vi "DriveExecute.vi"(8 "error in (no error)":errorcluster) -> (0 "error out":errorcluster)   [LabVIEW 2023]
doc: "Execute for Drie\n\nClosed control loop for drive\n\ninput: \n error in (cluster)\n\noutput:\n error out (cluster)"
uses:
  <vilib>/Rock Robotics/WPI/ThirdParty/JAS_Junk/TrajLib/LinearFilter_ResetToValue.vi
  <vilib>/Rock Robotics/WPI/ThirdParty/JAS_Junk/TrajLib/LinearFilter_Calculate.vi
  DriveGlobal.vi
  <vilib>/Rock Robotics/WPI/ThirdParty/JAS_Junk/TrajLib/LinearFilter_MovingAverage.vi
  <vilib>/Rock Robotics/WPI/ThirdParty/JAS_Junk/TrajLib/LinearFilter_LowPassBW1.vi
  <vilib>/Rock Robotics/WPI/ThirdParty/JAS_Junk/TrajLib/LinearFilter_LowPassBW2.vi
  <vilib>/Rock Robotics/WPI/ThirdParty/JAS_Junk/TrajLib/LinearFilter_HighPassBW1.vi
  <vilib>/Rock Robotics/WPI/ThirdParty/JAS_Junk/TrajLib/LinearFilter_HighPassBW2.vi
  <vilib>/Rock Robotics/WPI/ThirdParty/JAS_Junk/TrajLib/Trajectory_Library.lvlib
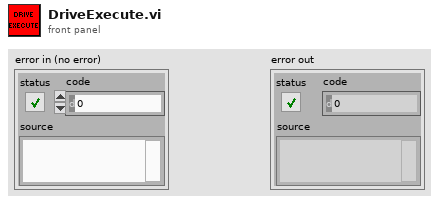
[diagram p1: front panel]
types:
  T1 = enum16{"Moving Average", "Low Pass 1st Order Butterworth", "Low Pass 2nd Order Butterworth", "High Pass 1st Order Butterworth", "High Pass 2nd Order Butterworth"}
  T2 = typedef "Trajectory_Library.lvlib/CHASSIS_SPEEDS.ctl" = cluster{"vX":dbl, "vY":dbl, "vOmega":dbl}
  T3 = typedef "ADIS16470 Device Reference.ctl" = cluster{"DevStatus":errorcluster, "Hardware Config":T4, "Calibration Complete":refnum<notifier>, "Status Reference":refnum<data-value>, "Data Reference":refnum<data-value>, "Sychronous Process VI":T8, "Cmd FIFO":refnum<k33>, "Source":T9, "Data FIFO":refnum<k33>, "Calibration Time (ms)":u32, "Data Reference":refnum<data-value>}
  T4 = typedef "ADIS16470 Hardware Configuration.ctl" = cluster{"SPI Clock Rate (Hz)":dbl, "IMU SPI Mode (3)":T5, "IMU Reset Pin":T6, "IMU SPI Bus":T7, "IMU Data Ready Pin":T6, "Stall Config":cluster{"Pow2BytesPerRead":u8, "StallTicks":u16, "CsToSclkTicks":u8}}
  T5 = typedef "WPI_SPIMode.ctl" = enum16{"Mode 0 (Clk Idle Low,Sample on Leading)", "Mode 1 (Clk Idle Low,Sample on Trailing)", "Mode 2 (Clk Idle High,Sample on Leading)", "Mode 3 (Clk Idle High,Sample on Trailing)"}
  T6 = typedef "FPGA_DIOChannel.ctl" = enum8{"DIO 0", "DIO 1", "DIO 2", "DIO 3", "DIO 4", "DIO 5", "DIO 6", "DIO 7", "DIO 8", "DIO 9", "DIO MXP 0", "DIO MXP 1", "DIO MXP 2", "DIO MXP 3", "DIO MXP 4", "DIO MXP 5", "DIO MXP 6", "DIO MXP 7", "DIO MXP 8", "DIO MXP 9", "DIO MXP 10", "DIO MXP 11", "DIO MXP 12", "DIO MXP 13", "DIO MXP 14", "DIO MXP 15", "SPI Port CS1", "SPI Port CS2", "SPI Port CS3", "SPI Port MISO", "SPI Port MOSI", "Invalid"}
  T7 = typedef "spi_bus.ctl" = enum16{"SPI On-Board, CS0", "SPI On-Board, CS1", "SPI On-Board, CS2", "SPI On-Board, CS3", "SPI MXP", "Invalid"}
  T8 = typedef "ADIS16470 Process.ctl" = refnum<vi>
  T9 = typedef "FPGA_CounterEncoderSourceConvertionLVSourceType.ctl" = cluster{"DevStatus":errorcluster, "AnalogTriggerMode?":bool, "DigitalMode":cluster{"DIO Channel":T10}, "AnalogTriggerMode":cluster{"AnalogTriggerIndex":T11, "OutputType":T12}}
  T10 = typedef "FPGA_DIODigitalSourceChannel.ctl" = enum8{"DIO 0", "DIO 1", "DIO 2", "DIO 3", "DIO 4", "DIO 5", "DIO 6", "DIO 7", "DIO 8", "DIO 9", "DIO MXP 0", "DIO MXP 1", "DIO MXP 2", "DIO MXP 3", "DIO MXP 4", "DIO MXP 5", "DIO MXP 6", "DIO MXP 7", "DIO MXP 8", "DIO MXP 9", "DIO MXP 10", "DIO MXP 11", "DIO MXP 12", "DIO MXP 13", "DIO MXP 14", "DIO MXP 15", "SPI Port CS1", "SPI Port CS2", "SPI Port CS3", "SPI Port MISO", "SPI Port MOSI", "Disabled"}
  T11 = typedef "FPGA_AnalogTriggerIndex.ctl" = enum8{"Trig 0", "Trig 1", "Trig 2", "Trig 3", "Trig 4", "Trig 5", "Trig 6", "Trig 7", "Invalid"}
  T12 = typedef "FPGA_AnalogTriggerOutType.ctl" = enum16{"InWindow", "TriggerState", "Rising", "Falling"}
  T13 = typedef "Trajectory_Library.lvlib/SWERVE_DRIVE_KINEMATICS.ctl" = cluster{"NumModules":i32, "InverseKinematics":T14, "ForwardKinematics":T14, "Modules":T15[], "PrevCoR":T15, "SavedModuleStates":T16[]}
  T14 = typedef "NI_Matrix.lvlib/RealMatrix.ctl" = dbl[][]
  T15 = typedef "Trajectory_Library.lvlib/TRANSLATION2D.ctl" = cluster{"X":dbl, "Y":dbl}
  T16 = typedef "Trajectory_Library.lvlib/SWERVE_DRIVE_MODULE_STATE.ctl" = cluster{"Speed":dbl, "Angle":T17}
  T17 = typedef "Trajectory_Library.lvlib/ROTATION2D.ctl" = cluster{"VALUE":dbl, "COS":dbl, "SIN":dbl}
  T18 = typedef "Trajectory_Library.lvlib/SWERVE_DRIVE_MODULE_POSITION.ctl" = cluster{"Distance":dbl, "Angle":T17, "P":bool}
  T19 = typedef "ADIS16470 Data.ctl" = cluster{"XAngle":dbl, "YAngle":dbl, "ZAngle":dbl}
  T20 = typedef "ADIS16470 Status.ctl" = cluster{"Calibrated?":bool, "IMU Detected?":bool}
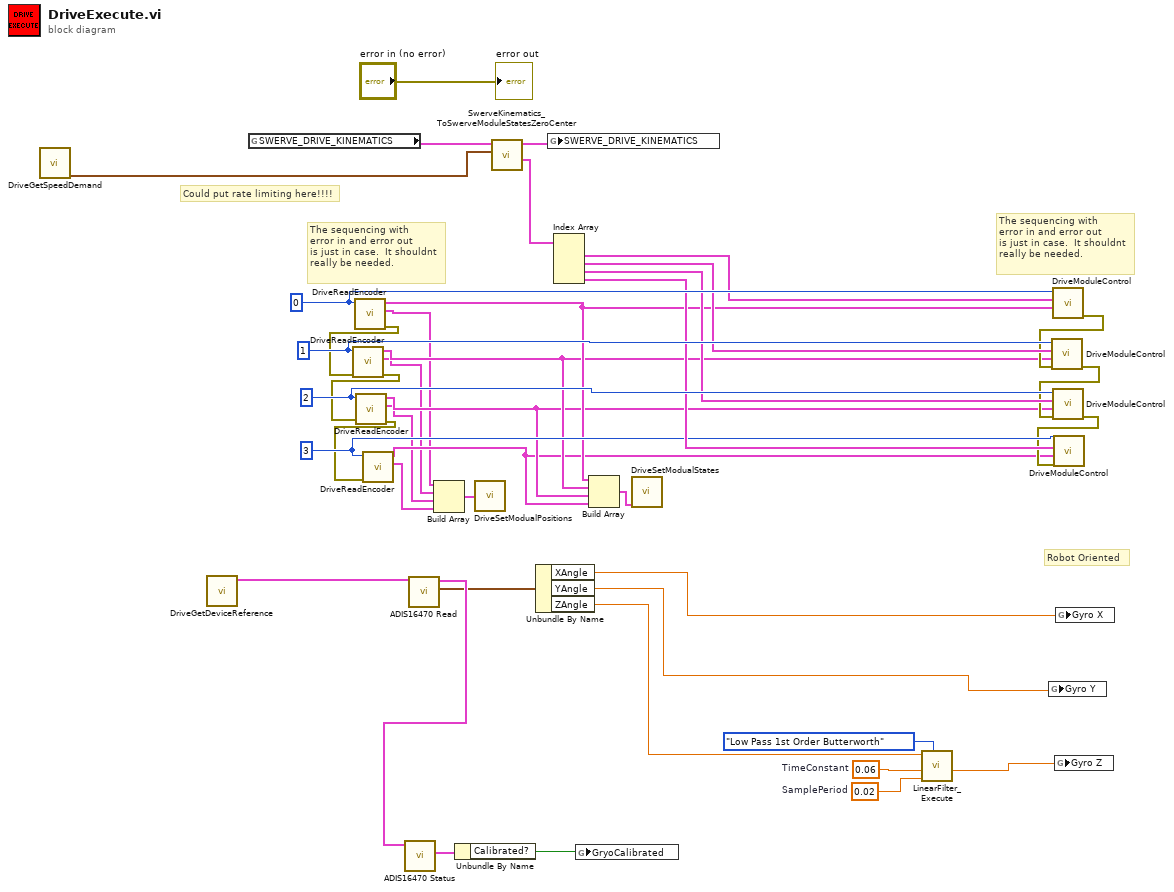
[diagram p0: block diagram]
diagram:
  w12 = 0.02  # SamplePeriod
  w11 = 0.06  # TimeConstant
  w37 = 0 ("ModualNamePrefix")
  w36 = 1 ("ModualNamePrefix")
  w35 = 2 ("ModualNamePrefix")
  w29 = 3 ("ModualNamePrefix")
  # "Robot Oriented"
  # "The sequencing with\nerror in and error out\nis just in case.  It shouldnt\nreally be needed."
  # "The sequencing with\nerror in and error out\nis just in case.  It shouldnt\nreally be needed."
  # "Could put rate limiting here!!!!"
  n1 = call "DriveGetSpeedDemand.vi"() -> ("ChassisSpeedDemand"=w39:T2)  [unwired: 8 in, 3 out]
  n2 = call "DriveGetDeviceReference.vi"() -> ("ADIS16470DevRef out"=w9:T3)  [unwired: 11 in]
  n3 = global read "DriveGlobal.vi" "SWERVE_DRIVE_KINEMATICS"() -> (w40:T13)
  n4 = call "DriveReadEncoder.vi"("ModualNamePrefix"=w37) -> ("error out"=w15:errorcluster, "SWERVE_DRIVE_MODULE_POSITION"=w21:T18, "SWERVE_DRIVE_MODULE_STATE"=w25:T16)  [unwired: 8 in]
  n5 = call "DriveReadEncoder.vi"("error in"=w15, "ModualNamePrefix"=w36) -> ("error out"=w14:errorcluster, "SWERVE_DRIVE_MODULE_POSITION"=w20:T18, "SWERVE_DRIVE_MODULE_STATE"=w24:T16)  [unwired: 7 in]
  n6 = call "DriveReadEncoder.vi"("error in"=w14, "ModualNamePrefix"=w35) -> ("error out"=w13:errorcluster, "SWERVE_DRIVE_MODULE_POSITION"=w19:T18, "SWERVE_DRIVE_MODULE_STATE"=w23:T16)  [unwired: 7 in]
  n7 = call "DriveReadEncoder.vi"("error in"=w13, "ModualNamePrefix"=w29) -> ("SWERVE_DRIVE_MODULE_POSITION"=w18:T18, "SWERVE_DRIVE_MODULE_STATE"=w22:T16)  [unwired: 7 in, 1 out]
  n8 = call <vilib>:"ADIS16470 Read.vi"("ADIS16470DevRef"=w9) -> ("ADIS16470 Value"=w5:T19, "ADIS16470DevRef"=w6:T3)  [unwired: 7 in, 2 out]
  n9 = call <vilib>:"ADIS16470 Status.vi"("ADIS16470DevRef"=w6) -> ("ADIS16470 Status"=w8:T20)  [unwired: 8 in, 2 out]
  n10 = Build Array(w21, w20, w19, w18) -> (w16:T18[])
  n11 = Unbundle By Name(w8) -> ("Calibrated?"=w7:bool)
  n12 = call "DriveSetModualPositions.vi"("Swerve_Drive_Modual_Position"=w16) -> ()  [unwired: 11 in]
  n13 = call <vilib>:"SwerveKinematics_ToSwerveModuleStatesZeroCenter.vi"("ChassisSpeeds"=w39, "in SWERVE_DRIVE_KINEMATICS"=w40) -> ("ModuleStates"=w34:T16[], "out SWERVE_DRIVE_KINEMATICS"=w38:T13)  [unwired: 8 in]
  n14 = Unbundle By Name(w5) -> ("XAngle"=w3:dbl, "YAngle"=w2:dbl, "ZAngle"=w4:dbl)
  n15 = global write "DriveGlobal.vi" "SWERVE_DRIVE_KINEMATICS"(w38) -> ()
  n16 = Index Array(array=w34) -> (element #1=w30:T16, element #2=w33:T16, element #3=w32:T16, element #4=w31:T16)  [unwired: 4 in]
  n17 = global write "DriveGlobal.vi" "GryoCalibrated"(w7) -> ()
  n18 = Build Array(w25, w24, w23, w22) -> (w17:T16[])
  n19 = call "DriveSetModualStates.vi"("Swerve__Drive_Modual_States"=w17) -> ()  [unwired: 11 in]
  n20 = call <vilib>:"LinearFilter_Execute.vi"("Filter Type"=T1."Low Pass 1st Order Butterworth", "SamplePeriod"=w12, "TimeConstant"=w11, "Input"=w4) -> ("Output"=w1:dbl)  [unwired: 6 in, 1 out]
  n21 = global write "DriveGlobal.vi" "Gyro Y"(w2) -> ()
  n22 = call "DriveModuleControl.vi"("Actual State"=w25, "Desired State"=w30, "ModualNamePrefix"=w37) -> ("error out"=w28:errorcluster)  [unwired: 8 in]
  n23 = call "DriveModuleControl.vi"("error in"=w28, "Actual State"=w24, "Desired State"=w33, "ModualNamePrefix"=w36) -> ("error out"=w27:errorcluster)  [unwired: 7 in]
  n24 = call "DriveModuleControl.vi"("error in"=w27, "Actual State"=w23, "Desired State"=w32, "ModualNamePrefix"=w35) -> ("error out"=w26:errorcluster)  [unwired: 7 in]
  n25 = call "DriveModuleControl.vi"("error in"=w26, "Actual State"=w22, "Desired State"=w31, "ModualNamePrefix"=w29) -> ()  [unwired: 7 in, 1 out]
  n26 = global write "DriveGlobal.vi" "Gyro Z"(w1) -> ()
  n27 = global write "DriveGlobal.vi" "Gyro X"(w3) -> ()
  "error out" <- "error in (no error)"
